vi "read station hall config noSCU.vi"(4 "name":string[](array[string])=["glass stall", "glass vent open", "glass flush close", "glass open", "sunshade stall", "sunshade flush close", "sunshade open ", "sunshade open 2", "vent open drift offset", "vent close drift offset", "glass open drift offset", "glass close drift offset", "sunshade open drift offset", "sunshade close drift offset", "sunshade open 2 drift offset", "sunshade close 2 drift offset"], 6 "section":string="Hall Counts", 8 "error in":errorcluster, 10 "default value":i32[](array[numeric]), 11 "configuration file path in":path) -> (0 "error out":errorcluster, 1 "Motor Drift Compensation":i32[](array[numeric])=[25, 25, 25, 25, 25, 25, 25, 25], 2 "Hall Positions":i32[](array[numeric]), 3 "configuration file path out":path)   [LabVIEW 2018]
uses:
  05.UserVI's/file io/ini/type defs/ini file actions.ctl
  05.UserVI's/file io/ini/type defs/ini entry types.ctl
  05.UserVI's/file io/ini/type defs/ini entry value.ctl
  05.UserVI's/file io/ini/type defs/ini entry.ctl
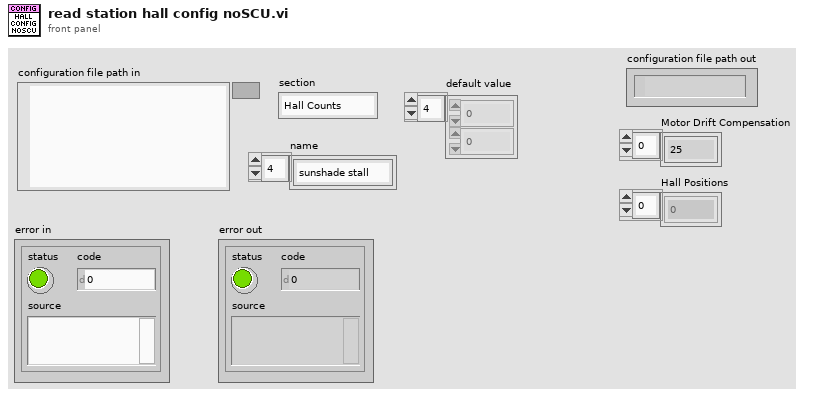
[diagram p1: front panel]
types:
  T1 = typedef "ini entry value.ctl" = cluster{"Boolean":bool, "Dbl":dbl, "I32":i32, "Path":path, "String":string, "U32":u32}
  T2 = typedef "ini entry types.ctl" = enum16{"Boolean", "Double", "I32", "Path", "String", "U32"}
  T3 = typedef "ini file actions.ctl" = enum16{"read ini", "write ini"}
  T4 = typedef "ini entry.ctl" = cluster{"section":string, "key":string, "type":T2, "default value":T1}
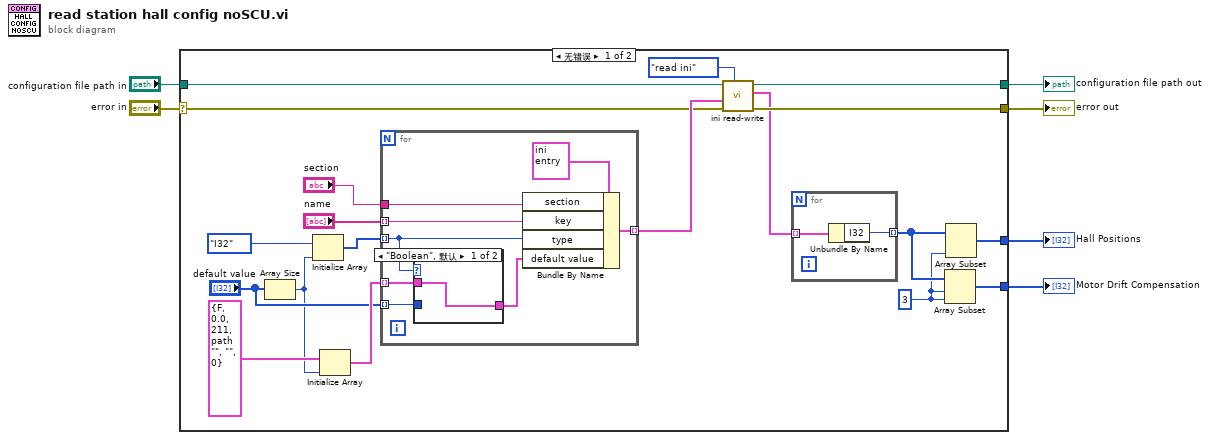
[diagram p0: block diagram]
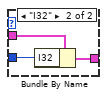
[diagram p2: hidden frame]
diagram:
  n1 = case shown="无错误" "error in" {
    selector: "error in" -> [w20 w41]
    tunnel: "configuration file path in" -> [w25 w40]
    tunnel: [w23 w40] -> w5
    tunnel: [w19 w41] -> w4
    tunnel: [w16 _] -> w2
    tunnel: [w15 _] -> w1
    frame No Error {
      w7 = 3
      n2 = Array Size(array="default value") -> (size(s)=w8:i32)
      n3 = Initialize Array(ini_entry_types."I32" ("type"), w8) -> (w12:T2[])
      n4 = Initialize Array(T1 {"Boolean"=FALSE, "Dbl"=0.0, "I32"=211, "Path"=path "", "String"="", "U32"=0} ("default value"), w8) -> (w10:T1[])
      n5 = for {
        tunnel: "section" -> [w34]
        tunnel: "name" -> [w33] mode=indexing
        tunnel: w12 -> [w31] mode=indexing
        tunnel: w10 -> [w30] mode=indexing
        tunnel: [w32] -> w21 mode=indexing
        tunnel: "default value" -> [w29] mode=indexing
        n6 = case shown="\"Boolean\", 默认" w31 {
          tunnel: w30 -> [w36 w39]
          tunnel: w29 -> [_ w38]
          tunnel: [w36 w37] -> w28
          frame "Boolean", Default {
          }
          frame "I32" {
            n7 = Bundle By Name(cluster=w39, "I32"=w38) -> (w37:T1)
          }
        }
        n8 = Bundle By Name(cluster=T4 {"section"="", "key"="", "type"=enum."Boolean", "default value"={"Boolean"=FALSE, "Dbl"=0.0, "I32"=0, "Path"=path "", "String"="", "U32"=0}}, "section"=w34, "key"=w33, "type"=w31, "default value"=w28) -> (w32:T4)
      }
      n9 = call "ini read-write.vi"("action"=ini_file_actions."read ini", "error in (no error)"=w20, "ini entry descriptors"=w21, "configuration file path"=w25) -> ("error out"=w19:errorcluster, "values out"=w18:T1[], "configuration file path out"=w23:path)  [unwired: 5 in]
      n10 = for {
        tunnel: w18 -> [w27] mode=indexing
        tunnel: [w26] -> w17 mode=indexing
        n11 = Unbundle By Name(w27) -> ("I32"=w26:i32)
      }
      n12 = Array Subset(array=w17, index=w7, length=w7) -> (w15:i32[])
      n13 = Array Subset(array=w17, length=w7) -> (w16:i32[])  [unwired: 1 in]
    }
    frame Error {
    }
  }
  "configuration file path out" <- w5
  "error out" <- w4
  "Hall Positions" <- w2
  "Motor Drift Compensation" <- w1
